vi "Frame Parcer.vi"(3 "Array":u8[](array[numeric])) -> ()   [LabVIEW 2016]
panel:
  out "Objects":T1(array[cluster])
  out "Number of Objects\nDetected":dbl
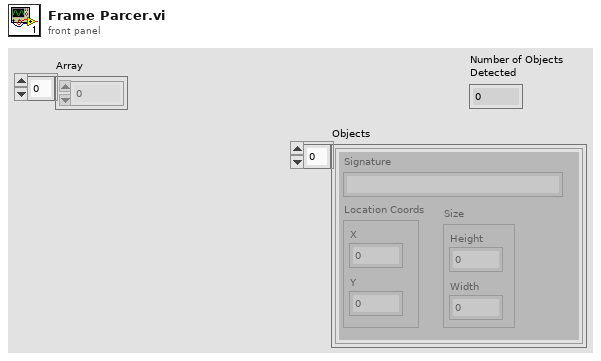
[diagram p1: front panel]
types:
  T1 = cluster{"Signature":string, "Location Coords":cluster{"X":dbl, "Y":dbl}, "Size":cluster{"Height":dbl, "Width":dbl}}[]
  T2 = cluster{"Signature":string, "Location Coords":cluster{"X":dbl, "Y":dbl}, "Size":cluster{"Height":dbl, "Width":dbl}}
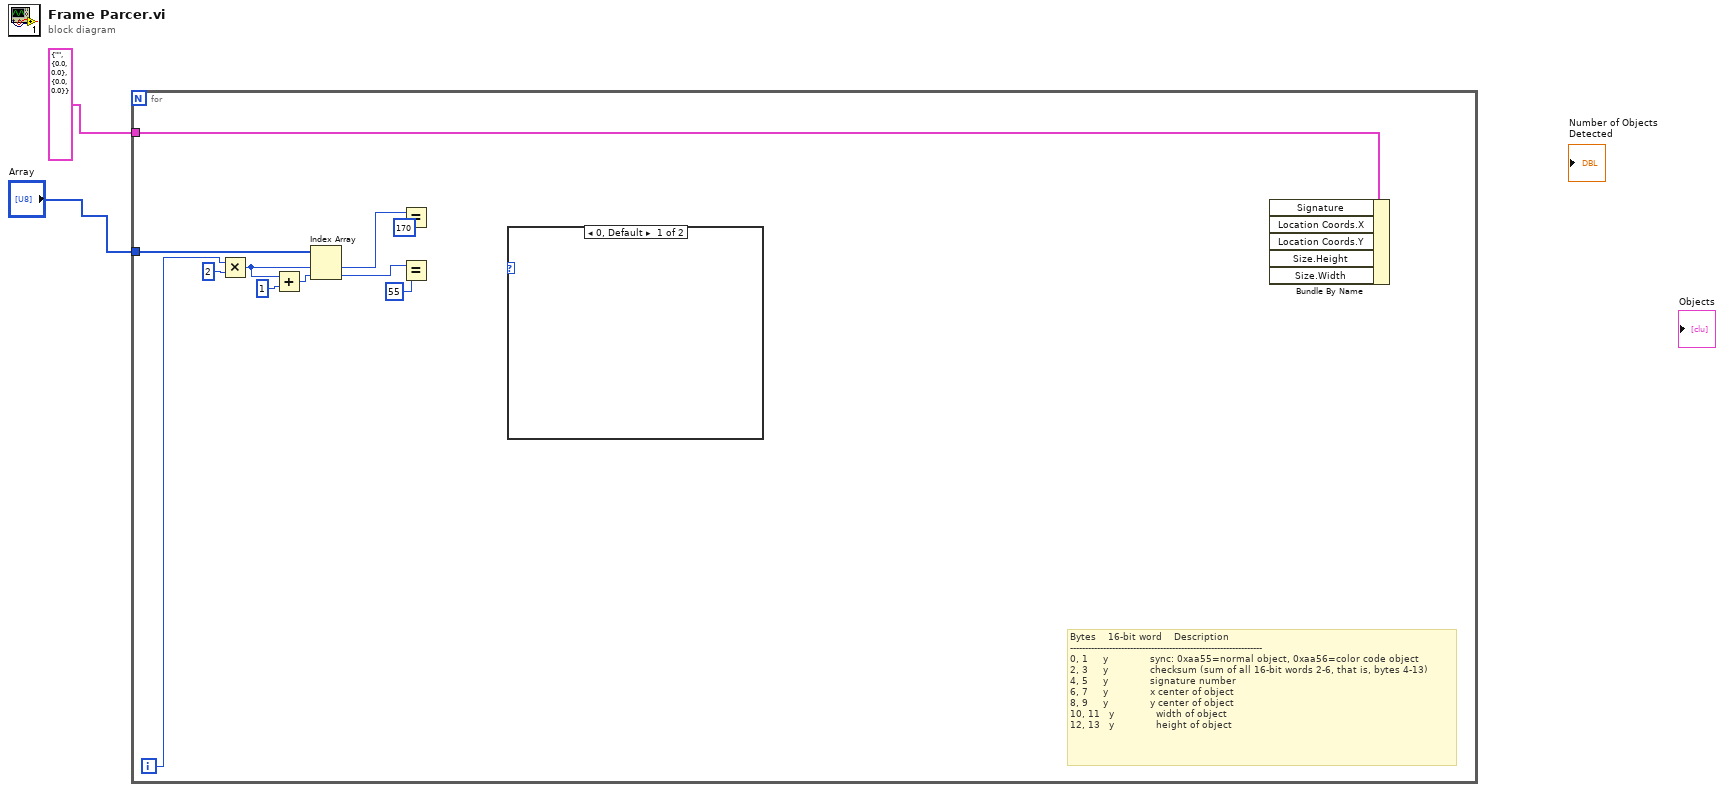
[diagram p0: block diagram]
diagram:
  n1 = for {
    tunnel: T2 {"Signature"="", "Location Coords"={"X"=0.0, "Y"=0.0}, "Size"={"Height"=0.0, "Width"=0.0}} ("Object Data") -> [w13]
    tunnel: "Array" -> [w12]
    i -> [w10]
    # "Bytes    16-bit word    Description\n----------------------------------------------------------------\n0, 1     y              sync: 0xaa55=normal object, 0xaa56=color code object\n2, 3     y              checksum (sum of all 16-bit words 2-6, that is, bytes 4-13)\n4, 5     y              signature number\n6, 7     y              x center of object\n8, 9     y              y center of object\n10, 11   y              width of object\n12, 13   y              height of object"
    n2 = Multiply(x=w10, y=2) -> (x*y=w8:i32)
    n3 = Add(x=w8, y=1) -> (x+y=w7:i32)
    n4 = Index Array(array=w12, index #1=w8, index #2=w7) -> (element #1=w6:u8, element #2=w5:u8)
    n5 = Equal?(x=w6, y=170) -> ()  [unwired: 1 out]
    n6 = Equal?(x=w5, y=55) -> ()  [unwired: 1 out]
    n7 = case shown="0, Default" {
      selector: _ -> [_ _]
      frame 0, Default {
      }
      frame 1 {
      }
    }
    n8 = Bundle By Name(cluster=w13) -> ()  [unwired: 5 in, 1 out]
  }
